vi "main.vi"() -> ()   [LabVIEW 2016]
uses:
  <vilib>/addons/_JKI Toolkits/Caraya/classes/Test Result/Node Results.ctl
  <vilib>/addons/_JKI Toolkits/Caraya/classes/Test Result/Test Node.ctl
  <vilib>/addons/_JKI Toolkits/Caraya/classes/Test Result/Test Registration Data.ctl
  <vilib>/addons/_JKI Toolkits/Caraya/classes/Test Result/Assert Event Data.ctl
  <vilib>/addons/_JKI Toolkits/Caraya/classes/Test Suite/Define Test Suite (Default).vi
  <vilib>/addons/_JKI Toolkits/Caraya/classes/Test Suite/Test Suite.lvclass
  <vilib>/addons/_JKI Toolkits/Caraya/classes/Test Result/Test Result.lvclass
panel:
  out "Test Results 2":T1[](array[typedef])
  in  "Run":bool
  in  "Stop":bool
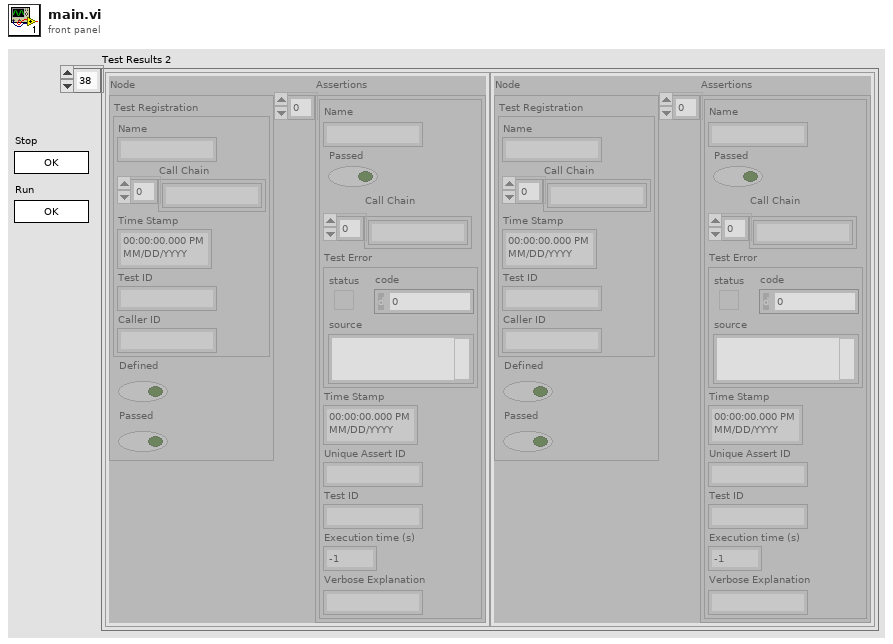
[diagram p1: front panel]
types:
  T1 = typedef "Caraya.lvlib/Test Result.lvclass/Node Results.ctl" = cluster{"Node":T2, "Assertions":T4[]}
  T2 = typedef "Caraya.lvlib/Test Result.lvclass/Test Node.ctl" = cluster{"Test Registration":T3, "Defined":bool, "Passed":bool}
  T3 = typedef "Caraya.lvlib/Test Result.lvclass/Test Registration Data.ctl" = cluster{"Name":string, "Call Chain":string[], "Time Stamp":timestamp, "Test ID":string, "Caller ID":string}
  T4 = typedef "Caraya.lvlib/Test Result.lvclass/Assert Event Data.ctl" = cluster{"Name":string, "Passed":bool, "Call Chain":string[], "Test Error":errorcluster, "Time Stamp":timestamp, "Unique Assert ID":string, "Test ID":string, "Execution time (s)":dbl, "Verbose Explanation":string}
  T5 = typedef "Caraya.lvlib/Test Suite.lvclass/Suite PublicEvents -- cluster.ctl" = cluster{"Test Suite Result Event":refnum<user-event>, "suite destroyed":refnum<user-event>}
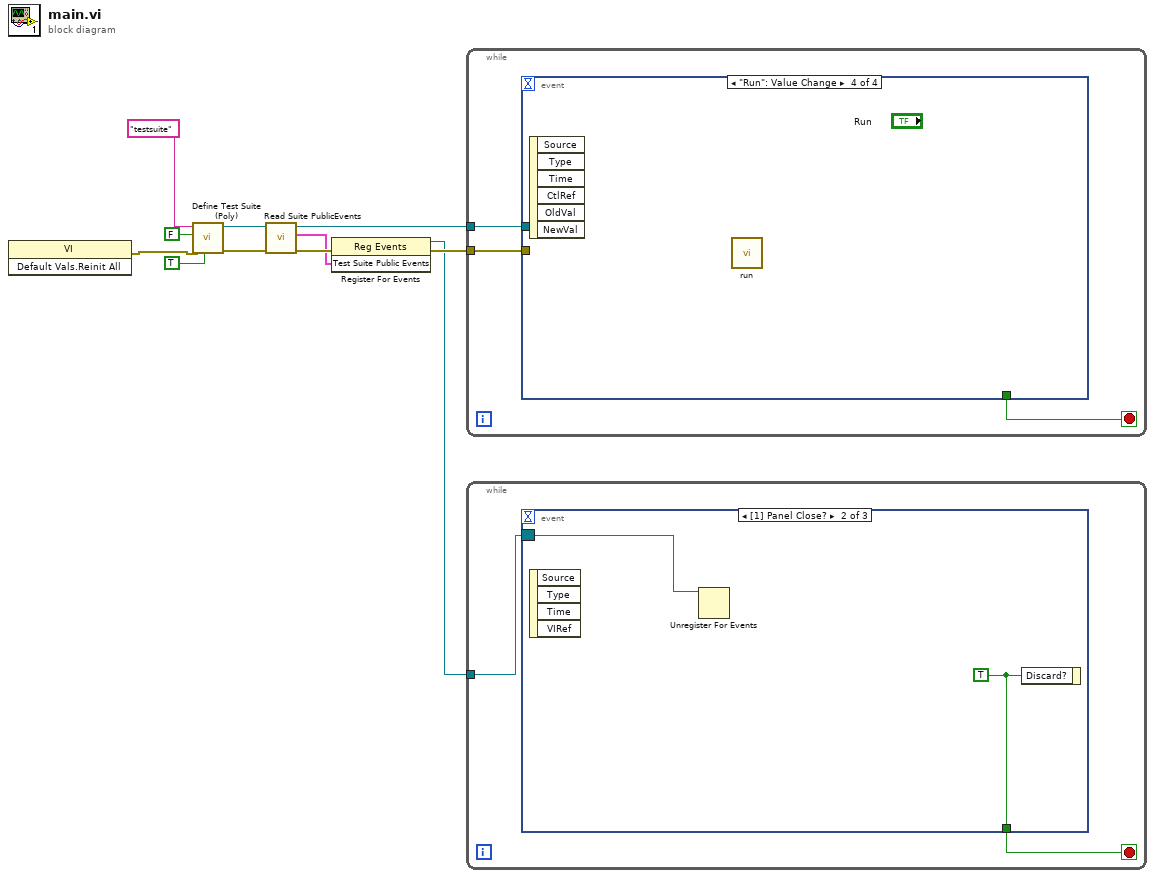
[diagram p0: block diagram]
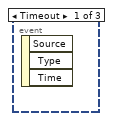
[diagram p2: hidden frame]
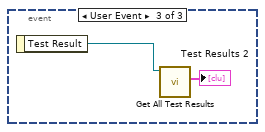
[diagram p3: hidden frame]
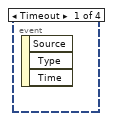
[diagram p4: hidden frame]
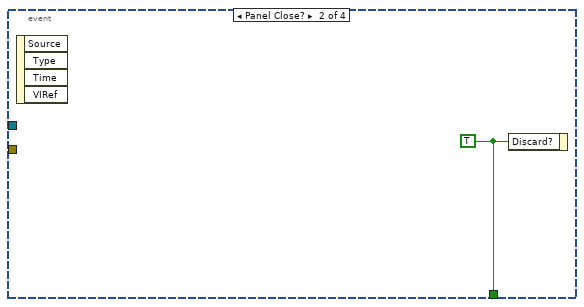
[diagram p5: hidden frame]
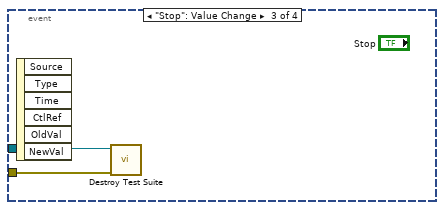
[diagram p6: hidden frame]
diagram:
  n1 = invoke class="VI" method="Default Vals.Reinit All"() -> (error out=w1:errorcluster)  [unwired: 3 in, 2 out]
  n2 = call-poly <vilib>:"Define Test Suite (Poly).vi"("Verbose (F)"=TRUE, "error in (no error)"=w1, "Interactive"=FALSE, "Label (VI Title)"="testsuite") -> ("error out"=w10:errorcluster, "Test Suite"=w11:refnum<class "Test Suite.lvclass">)  [unwired: 6 in]
  n3 = call <vilib>:"Read Suite PublicEvents.vi"("error in (no error)"=w10, "Test Suite in"=w11) -> ("error out"=w8:errorcluster, "Test Suite Public Events"=w6:T5, "Test Suite out"=w9:refnum<class "Test Suite.lvclass">)  [unwired: 7 in]
  n4 = register-events(error in=w8, w6) -> (reference out=w2:refnum<event-registration>, error out=w7:errorcluster)  [unwired: 1 in]
  n5 = while {
    tunnel: w9 -> [w14]
    tunnel: w7 -> [w13]
    stop <- w12 stop-if-true
    n6 = event shown="[3] \"Run\": Value Change" {
      selector: _ -> [_ _ _ _]
      dyn-events: _ -> [_ _ _ _]
      timeout: _ -> [_ _ _ _]
      tunnel: w14 -> [_ _ w17 _]
      tunnel: w13 -> [_ _ w16 _]
      tunnel: [_ w15 _ _] -> w12
      event Timeout {
        n7 = event-data() -> ()  [unwired: 1 in, 3 out]
      }
      event Panel Close? {
        w15 = TRUE ("Discard?")
        n8 = event-data() -> ()  [unwired: 1 in, 4 out]
        n9 = event-data("Discard?"=w15) -> ()  [unwired: 1 in, 1 out]
      }
      event "Stop": Value Change {
        n10 = event-data() -> ()  [unwired: 1 in, 6 out]
        n11 = call-dynamic "Destroy Test Suite.vi"("error in (no error)"=w16, "Test Suite in"=w17) -> ()  [unwired: 8 in, 2 out]
      }
      event "Run": Value Change {
        n12 = event-data() -> ()  [unwired: 1 in, 6 out]
        n13 = call "run.vi"() -> ()  [unwired: 12 in]
      }
    }
  }
  n14 = while {
    tunnel: w2 -> [w18]
    stop <- w19 stop-if-true
    n15 = event shown="[1] Panel Close?" {
      selector: w18 -> [_ w20 _]
      dyn-events: _ -> [_ _ _]
      timeout: _ -> [_ _ _]
      tunnel: [_ w21 _] -> w19
      event Timeout {
        n16 = event-data() -> ()  [unwired: 1 in, 3 out]
      }
      event Panel Close? {
        w21 = TRUE ("Discard?")
        n17 = event-data() -> ()  [unwired: 1 in, 4 out]
        n18 = Unregister For Events(event registration refnum=w20) -> ()  [unwired: 1 in, 1 out]
        n19 = event-data("Discard?"=w21) -> ()  [unwired: 1 in, 1 out]
      }
      event User Event {
        n20 = event-data() -> ("Test Result"=w23:refnum<class "Test Result.lvclass">)  [unwired: 1 in]
        n21 = call <vilib>:"Get All Test Results.vi"("Test Result in"=w23) -> ("Test Results"=→"Test Results 2":T1[])  [unwired: 8 in, 2 out]
      }
    }
  }
